vi "8.2.vi"() -> ()   [LabVIEW 2017]
panel:
  out "sum":i32
  out "variant":variant
  out "G":string
  out "B":string
  out "E":string
  out "D":string
  out "C":string
  out "F":string
  out "A":string
  out "Numeric 2":i32
  out "Numeric":i32
  out "subarray":string[](array[string])
  in  "String":string="be cfbegad cbdgef fgaecd cgeb fdcge agebfd fecdb fabcd edb | fdgacbe cefdb cefbgd gcbe\nedbfga begcd cbg gc gcadebf fbgde acbgfd abcde gfcbed gfec | fcgedb cgb dgebacf gc\nfgaebd cg bdaec gdafb agbcfd gdcbef bgcad gfac gcb cdgabef | cg cg fdcagb cbg\nfbegcd cbd adcefb dageb afcb bc aefdc ecdab fgdeca fcdbega | efabcd cedba gadfec cb\naecbfdg fbg gf bafeg dbefa fcge gcbea fcaegb dgceab fcbdga | gecf egdcabf bgf bfgea\nfgeab ca afcebg bdacfeg cfaedg gcfdb baec bfadeg bafgc acf | gebdcfa ecba ca fadegcb\ndbcfg fgd bdegcaf fgec aegbdf ecdfab fbedc dacgb gdcebf gf | cefg dcbef fcge gbcadfe\nbdfegc cbegaf gecbf dfcage bdacg ed bedf ced adcbefg gebcd | ed bcgafe cdgba cbgef\negadfb cdbfeg cegd fecab cgb gbdefca cg fgcdab egfdb bfceg | gbdfcae bgc cg cgb\ngcafb gcf dcaebfg ecagb gf abcdeg gaef cafbge fdbac fegbdc | fgae cfgab fg bagce"
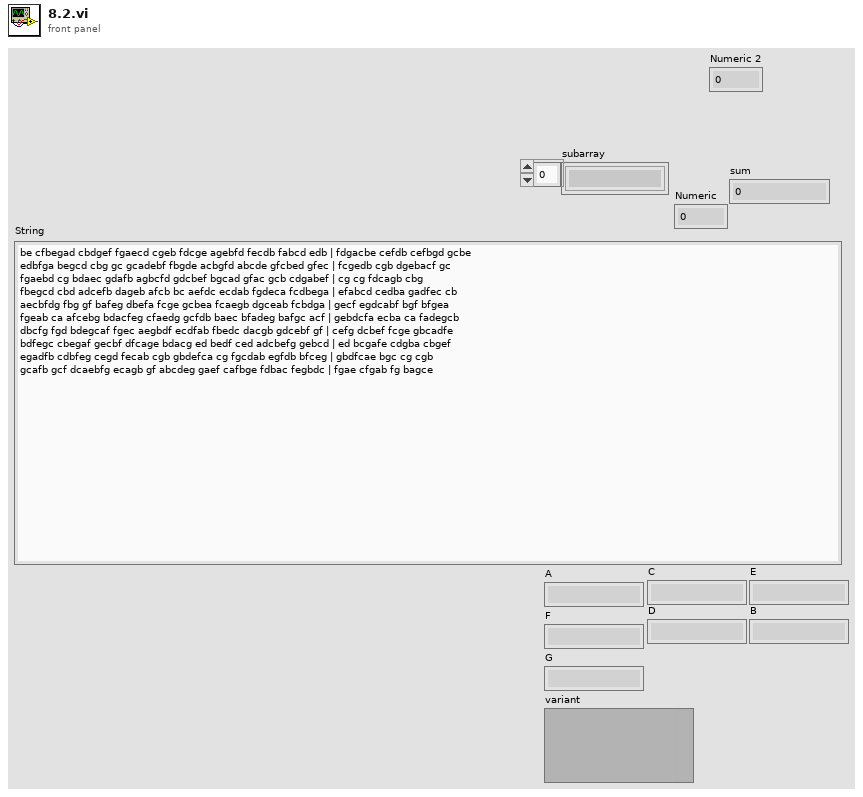
[diagram p1: front panel]
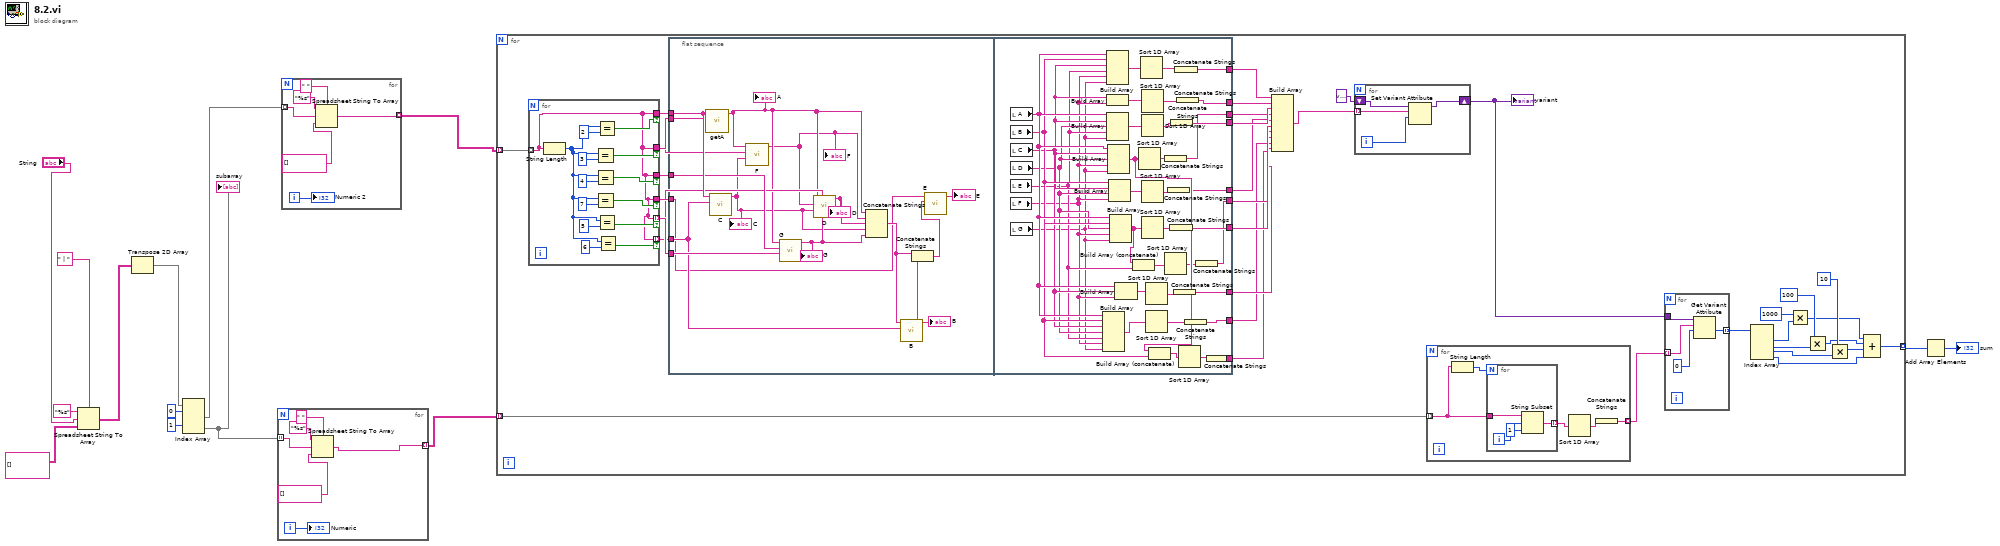
[diagram p0: block diagram]
diagram:
  n1 = Spreadsheet String To Array(delimiter (Tab)=" | ", format string="%s", spreadsheet string="String", array type (2D Dbl)=string[][] []) -> (array=w10:string[][])
  n2 = Transpose 2D Array(2D array=w10) -> (transposed array=w9:string[][])
  n3 = Index Array(array=w9, index (row) #1=0 ("index (row)"), index (row) #2=1 ("index (row)")) -> (element #1=w5:string[], element #2=w7:string[])  [unwired: 2 in]
  "subarray" <- w7
  n4 = for {
    tunnel: w7 -> [w20] mode=indexing
    tunnel: [w15] -> w3 mode=indexing
    i -> [w16]
    n5 = Spreadsheet String To Array(delimiter (Tab)=" ", format string="%s", spreadsheet string=w20, array type (2D Dbl)=string[] []) -> (array=w15:string[])
    "Numeric" <- w16
  }
  n6 = for {
    tunnel: w5 -> [w26] mode=indexing
    tunnel: [w21] -> w4 mode=indexing
    i -> [w22]
    n7 = Spreadsheet String To Array(delimiter (Tab)=" ", format string="%s", spreadsheet string=w26, array type (2D Dbl)=string[] []) -> (array=w21:string[])
    "Numeric 2" <- w22
  }
  n8 = for {
    tunnel: w4 -> [w60] mode=indexing
    tunnel: w3 -> [w41] mode=indexing
    tunnel: [w27] -> w2 mode=indexing
    n9 = for {
      tunnel: w60 -> [w131] mode=indexing
      tunnel: [w131] -> w59 if=w136
      tunnel: [w131] -> w58 if=w135
      tunnel: [w131] -> w57 if=w134
      tunnel: [w131] -> w54 if=w133
      tunnel: [w131] -> w56 mode=indexing if=w132
      tunnel: [w131] -> w55 mode=indexing if=w130
      n10 = String Length(string=w131) -> (length=w137:i32)
      n11 = Equal?(x=w137, y=3) -> (x = y?=w135:bool)
      n12 = Equal?(x=w137, y=4) -> (x = y?=w134:bool)
      n13 = Equal?(x=w137, y=7) -> (x = y?=w133:bool)
      n14 = Equal?(x=w137, y=2) -> (x = y?=w136:bool)
      n15 = Equal?(x=w137, y=5) -> (x = y?=w132:bool)
      n16 = Equal?(x=w137, y=6) -> (x = y?=w130:bool)
    }
    n17 = flat-sequence {
      tunnel: w59 -> [w88]
      tunnel: w58 -> [w87]
      tunnel: w57 -> [w86]
      tunnel: w56 -> [w85]
      tunnel: w55 -> [w81]
      tunnel: w54 -> [w74]
      tunnel: [w106] -> w52
      tunnel: [w105] -> w51
      tunnel: [w104] -> w50
      tunnel: [w103] -> w49
      tunnel: [w102] -> w48
      tunnel: [w101] -> w47
      tunnel: [w100] -> w46
      tunnel: [w99] -> w45
      tunnel: [w98] -> w44
      tunnel: [w97] -> w43
      frame #0 {
        n18 = call "getA.vi"("format string"=w87, "format string 2"=w88) -> ("result string"=w84:string)  [unwired: 9 in]
        "A" <- w84
        n19 = call "C.vi"("6"=w81, "CF"=w88) -> ("C"=w76:string)  [unwired: 9 in]
        "C" <- w76
        n20 = call "F.vi"("String"=w76, "format string"=w87, "result string in"=w84) -> ("result string out"=w77:string)  [unwired: 8 in]
        "F" <- w77
        n21 = call "G.vi"("5"=w85, "4"=w86, "A"=w84) -> ("G"=w82:string)  [unwired: 8 in]
        "G" <- w82
        n22 = call "D.vi"("G"=w82, "5"=w85, "C"=w76, "F"=w77, "A"=w84) -> ("D"=w83:string)  [unwired: 6 in]
        "D" <- w83
        n23 = Concatenate Strings(w84, w77, w83, w76, w82) -> (w80:string)
        n24 = call "B.vi"("Array"=w81, "String"=w80) -> ("B"=w79:string)  [unwired: 9 in]
        "B" <- w79
        n25 = Concatenate Strings(w80, w79) -> (w78:string)
        n26 = call "E.vi"("String"=w78, "format string in"=w74) -> ("format string out"=→"E":string)  [unwired: 9 in]
      }
      frame #1 {
        n27 = local read "A"() -> (w96:string)
        n28 = local read "B"() -> (w95:string)
        n29 = local read "C"() -> (w94:string)
        n30 = local read "D"() -> (w93:string)
        n31 = local read "E"() -> (w92:string)
        n32 = local read "F"() -> (w91:string)
        n33 = local read "G"() -> (w90:string)
        n34 = Build Array(w96, w95, w94, w93, w92, w91, w90) -> (w89:string[])
        n35 = Build Array(w96, w95, w94, w92, w91, w90) -> (w125:string[])
        n36 = Build Array(w94, w91) -> (w124:string[])
        n37 = Build Array(w96, w94, w93, w92, w90) -> (w123:string[])
        n38 = Build Array(w96, w94, w93, w91, w90) -> (w118:string[])
        n39 = Build Array(w95, w94, w93, w91) -> (w122:string[])
        n40 = Build Array(w96, w95, w93, w91, w90) -> (w121:string[])
        n41 = Build Array(w96, w94, w91) -> (w119:string[])
        n42 = Build Array (concatenate)(w121, w92) -> (w120:string[])
        n43 = Sort 1D Array(array=w118) -> (sorted array=w113:string[])
        n44 = Sort 1D Array(array=w125) -> (sorted array=w116:string[])
        n45 = Sort 1D Array(array=w124) -> (sorted array=w115:string[])
        n46 = Sort 1D Array(array=w123) -> (sorted array=w114:string[])
        n47 = Sort 1D Array(array=w122) -> (sorted array=w112:string[])
        n48 = Sort 1D Array(array=w121) -> (sorted array=w111:string[])
        n49 = Sort 1D Array(array=w119) -> (sorted array=w109:string[])
        n50 = Sort 1D Array(array=w89) -> (sorted array=w108:string[])
        n51 = Build Array (concatenate)(w118, w95) -> (w117:string[])
        n52 = Concatenate Strings(w113) -> (w103:string)
        n53 = Sort 1D Array(array=w120) -> (sorted array=w110:string[])
        n54 = Concatenate Strings(w112) -> (w102:string)
        n55 = Concatenate Strings(w111) -> (w101:string)
        n56 = Concatenate Strings(w114) -> (w104:string)
        n57 = Concatenate Strings(w109) -> (w99:string)
        n58 = Concatenate Strings(w116) -> (w106:string)
        n59 = Concatenate Strings(w115) -> (w105:string)
        n60 = Sort 1D Array(array=w117) -> (sorted array=w107:string[])
        n61 = Concatenate Strings(w108) -> (w98:string)
        n62 = Concatenate Strings(w110) -> (w100:string)
        n63 = Concatenate Strings(w107) -> (w97:string)
      }
    }
    n64 = Build Array(w52, w51, w50, w49, w48, w47, w46, w45, w44, w43) -> (w42:string[])
    n65 = for {
      tunnel: w42 -> [w128] mode=indexing
      shift-right: [w127] -> w39
      shift-left: variant ("variant") -> [w126]
      i -> [w129]
      n66 = Set Variant Attribute(Variant=w126, name=w128, value=w129) -> (Variant out=w127:variant)  [unwired: 1 in, 2 out]
    }
    "variant" <- w39
    n67 = for {
      tunnel: w41 -> [w68] mode=indexing
      tunnel: [w65] -> w40 mode=indexing
      n68 = String Length(string=w68) -> (length=w69:i32)
      n69 = for {
        N: w69 -> [_]
        tunnel: w68 -> [w73]
        tunnel: [w70] -> w67 mode=indexing
        i -> [w72]
        n70 = String Subset(string=w73, offset (0)=w72, length (rest)=1 ("length (rest)")) -> (substring=w70:string)
      }
      n71 = Sort 1D Array(array=w67) -> (sorted array=w66:string[])
      n72 = Concatenate Strings(w66) -> (w65:string)
    }
    n73 = for {
      tunnel: w40 -> [w63] mode=indexing
      tunnel: w39 -> [w64]
      tunnel: [w61] -> w38 mode=indexing
      n74 = Get Variant Attribute(Variant=w64, name=w63, default value (empty Variant)=0) -> (value=w61:i32)  [unwired: 1 in, 3 out]
    }
    n75 = Index Array(array=w38) -> (element #1=w37:i32, element #2=w36:i32, element #3=w35:i32, element #4=w28:i32)  [unwired: 4 in]
    n76 = Multiply(x=1000, y=w37) -> (x*y=w31:i32)
    n77 = Multiply(x=100, y=w36) -> (x*y=w30:i32)
    n78 = Multiply(x=10, y=w35) -> (x*y=w29:i32)
    n79 = Compound Arithmetic op=ADD(w31, w30, w29, w28) -> (w27:i32)
  }
  n80 = Add Array Elements(numeric array=w2) -> (sum=→"sum":i32)
